vi "MultiPlane.vi"(0 "Digitizer Settings":T5={"Digitizer delay (us) "=0.0, "rf points per line"=2048, "lines per plane"=128, "Samp Rate (Hz)"=100000000.0, "Additional dig delay (us)"=0.0, "Voltage Scale"=0.4, "Pre-Looks"=0, "Offset delay (us)"=0.0, "bits A/D"=8, "Avg Num"=1, "DigTimeOut"=5.0, "Rel Dig Delay"=0.0, "Dig Ch"=0, "LeCroyCluster"={"LeCroy Channels"=[TRUE, FALSE, FALSE, FALSE], "LC read pt offset"=0.0, "Sweep Avg"=FALSE}, "Main Digitizer"=enum."NI Digitizer", "Dig Config"=enum."Single channel", "Digitizer ID Cluster"={"Acqiris/Alazar/SP ID"=[], "NI Instr Handles"=[], "LeCroy VISA"="", "GaGe Handle"={"Handle"=0, "Sample size"=0, "Resolution"=0, "Offset"=0, "Channels"=0, "Boards"=0}, "ATS Ref"="ATS9350", "Acqiris Address"=["PCI::INSTR0"], "ADQRef"=refnum, "adq_cu_ptr"=refnum}, "Trigger Settings"={"Trig Source"=1, "Trig Coupling"=0, "Trig Slope"=0, "Level (mV)"=1500.0}, "Bulk Acq"=FALSE, "Bulk Start Indexes"=[], "Data Ref RF"=refnum, "NI ID/Channel"=[], "Total Dig CH"=5, "Xtra Ann Trig delay (us)"=10.0, "Fix Z Delay?"=FALSE, "One Way Transmission?"=FALSE, "Data Ref Log"=refnum} {"Trigger Settings"."Trig Slope" items=["Positive", "Negative"]; "Trigger Settings"."Level (mV)" format="%.2f"; "Trigger Settings"."Trig Coupling" items=["DC 1 MOhm", "AC 1 MOhm", "DC 50 Ohm", "AC 50 Ohm"]; "Trigger Settings"."Trig Source" items=["Chan 1", "External"]; "Rel Dig Delay" format="%.2f"; "DigTimeOut" format="%.2f"; "Avg Num" min=1; "Offset delay (us)" format="%.2f"; "Additional dig delay (us)" format="%.2f"; "Digitizer delay (us)" format="%.2f"}, 1 "Scan data":T9 {"axis 2 ticks" format="%.2f"; "axis 1 ticks" format="%.2f"; "step size" format="%.2f"; "axis2o" format="%.2f"; "axis1o" format="%.2f"; "Pulse Parameters"."pos peak pressure (MPa)" format="%.2f"; "Pulse Parameters"."focal length (cm)" format="%.2f"; "Pulse Parameters"."MI" format="%.2f"; "Pulse Parameters"."Ita.3" format="%.2f"; "Pulse Parameters"."Temporal Av Intensity \n(Ita mW/cm^2)" format="%.2f"; "Pulse Parameters"."Ipa.3" format="%.2f"; "Pulse Parameters"."Pulse Av Intensity\n (Ipa W/cm^2)" format="%.2f"; "Pulse Parameters"."Pulse Int \nIntegral (PII J/cm^2)" format="%.2f"; "Pulse Parameters"."pulse dur (Pd s)" format="%.2f"; "Pulse Parameters"."p.3" format="%.2f"; "Pulse Parameters"."neg peak pressure (MPa)" format="%.2f"; "Pulse Parameters"."derating (.3) factor" format="%.2f"; "Pulse Parameters"."prf" format="%.2f"; "Pulse Parameters"."Frequency (MHz)" format="%.2f"; "scan data" format="%.2f"}, 3 "Number of z planes":i32=1, 5 "Parameter Selection":u16, 6 "Dig delay":dbl, 7 "Motion Settings":T1={"No Motion?"=FALSE, "Motion System"=enum."No Motion Card", "Motion Bd ID"=1, "Motion Profile"="SMAC1", "# Axis"=1, "Reverse Z axis?"=TRUE, "SMAC Axis"=0, "scan pair"=enum."y-(x) scan", "RT fps"=6.0, "Steps per mm"=[1000, 1000, 1000, 1000], "Motor Parameters"={"velocity ct/s"=[10000.0, 10000.0, 10000.0, 50000.0], "accel ct/s^2"=[50000.0, 50000.0, 50000.0, 200000.0]}, "One Way Scan"=FALSE, "Reverse One Way Scan"=FALSE, "Global Position (mm)"=[], "Plane"=0, "Distance between\nscan lines (um)"=0.0, "Distance between\nscan planes (um)"=0.0, "number of scan planes"=1, "Total steps in line"=0, "Xtra plane\ndistance  (um)"=100, "Xtra planes "=1, "Add Axis"=FALSE, "overshoot cts"=200, "BKPT Shift"=0, "Scan Start Time (ms)"=0, "ESP VISA"="GPIB::1::INSTR", "3rd Axis"=1, "GL Ref Out"=refnum, "Galil Address"=""} {"3rd Axis" items=["x", "y", "z", "w"]; "Xtra planes" min=1; "Xtra plane\ndistance  (um)" min=0; "Distance between\nscan planes (um)" format="%.2f"; "Distance between\nscan lines (um)" format="%.2f"; "SMAC Axis" items=["None"=0, "Axis 1"=1, "Axis 2"=2, "Axis 3"=3, "Axis 4"=4, "Axis 5"=5, "Axis 6"=6, "Axis 7"=7, "Axis 8"=8, "Vector Space 1"=17, "Vector Space 2"=18, "Vector Space 3"=19, "Vector Space 4"=20]; "Motion Bd ID" min=1 max=32 step=1}, 9 "Current plane":i32, 11 "z plane spacing":i32, 12 "file name":string) -> (4 "Digitizer Settings Out":T5={"Digitizer delay (us) "=0.0, "rf points per line"=2048, "lines per plane"=128, "Samp Rate (Hz)"=100000000.0, "Additional dig delay (us)"=0.0, "Voltage Scale"=0.4, "Pre-Looks"=0, "Offset delay (us)"=0.0, "bits A/D"=8, "Avg Num"=1, "DigTimeOut"=5.0, "Rel Dig Delay"=0.0, "Dig Ch"=0, "LeCroyCluster"={"LeCroy Channels"=[TRUE, FALSE, FALSE, FALSE], "LC read pt offset"=0.0, "Sweep Avg"=FALSE}, "Main Digitizer"=enum."NI Digitizer", "Dig Config"=enum."Single channel", "Digitizer ID Cluster"={"Acqiris/Alazar/SP ID"=[], "NI Instr Handles"=[], "LeCroy VISA"="", "GaGe Handle"={"Handle"=0, "Sample size"=0, "Resolution"=0, "Offset"=0, "Channels"=0, "Boards"=0}, "ATS Ref"="ATS9350", "Acqiris Address"=["PCI::INSTR0"], "ADQRef"=refnum, "adq_cu_ptr"=refnum}, "Trigger Settings"={"Trig Source"=1, "Trig Coupling"=0, "Trig Slope"=0, "Level (mV)"=1500.0}, "Bulk Acq"=FALSE, "Bulk Start Indexes"=[], "Data Ref RF"=refnum, "NI ID/Channel"=[], "Total Dig CH"=5, "Xtra Ann Trig delay (us)"=10.0, "Fix Z Delay?"=FALSE, "One Way Transmission?"=FALSE, "Data Ref Log"=refnum} {"Trigger Settings"."Trig Slope" items=["Positive", "Negative"]; "Trigger Settings"."Level (mV)" format="%.2f"; "Trigger Settings"."Trig Coupling" items=["DC 1 MOhm", "AC 1 MOhm", "DC 50 Ohm", "AC 50 Ohm"]; "Trigger Settings"."Trig Source" items=["Chan 1", "External"]; "Rel Dig Delay" format="%.2f"; "DigTimeOut" format="%.2f"; "Avg Num" min=1; "Offset delay (us)" format="%.2f"; "Additional dig delay (us)" format="%.2f"; "Digitizer delay (us)" format="%.2f"}, 15 "Motion Settings Out":T1={"No Motion?"=FALSE, "Motion System"=enum."No Motion Card", "Motion Bd ID"=1, "Motion Profile"="SMAC1", "# Axis"=1, "Reverse Z axis?"=TRUE, "SMAC Axis"=0, "scan pair"=enum."y-(x) scan", "RT fps"=6.0, "Steps per mm"=[1000, 1000, 1000, 1000], "Motor Parameters"={"velocity ct/s"=[10000.0, 10000.0, 10000.0, 50000.0], "accel ct/s^2"=[50000.0, 50000.0, 50000.0, 200000.0]}, "One Way Scan"=FALSE, "Reverse One Way Scan"=FALSE, "Global Position (mm)"=[], "Plane"=0, "Distance between\nscan lines (um)"=0.0, "Distance between\nscan planes (um)"=0.0, "number of scan planes"=1, "Total steps in line"=0, "Xtra plane\ndistance  (um)"=100, "Xtra planes "=1, "Add Axis"=FALSE, "overshoot cts"=200, "BKPT Shift"=0, "Scan Start Time (ms)"=0, "ESP VISA"="GPIB::1::INSTR", "3rd Axis"=1, "GL Ref Out"=refnum, "Galil Address"=""} {"3rd Axis" items=["x", "y", "z", "w"]; "Xtra planes" min=1; "Xtra plane\ndistance  (um)" min=0; "Distance between\nscan planes (um)" format="%.2f"; "Distance between\nscan lines (um)" format="%.2f"; "SMAC Axis" items=["None"=0, "Axis 1"=1, "Axis 2"=2, "Axis 3"=3, "Axis 4"=4, "Axis 5"=5, "Axis 6"=6, "Axis 7"=7, "Axis 8"=8, "Vector Space 1"=17, "Vector Space 2"=18, "Vector Space 3"=19, "Vector Space 4"=20]; "Motion Bd ID" min=1 max=32 step=1})   [LabVIEW 2022 SP3]
uses:
  ScanningControl/Digitizers/-DigitizerRoutines/DigitizerSettings.ctl
  ScanningControl/Digitizers/-DigitizerRoutines/Digitizer.ctl
  ScanningControl/Digitizers/-DigitizerRoutines/DigConfig.ctl
  ScanningControl/Digitizers/-DigitizerRoutines/DigitizerID.ctl
  C:/Windows/System32/ADQAPI_dotNet_helper.dll
  ScanningControl/Motion Controllers/NI_controller/-NI_MotionRoutines/MotionParameters.ctl
  ScanningControl/Motion Controllers/NI_controller/-NI_MotionRoutines/MotionSys.ctl
  ScanningControl/Motion Controllers/-MotionRoutines/ScanAxis.ctl
  ScanningControl/Motion Controllers/-MotionRoutines/3rdAxis.ctl
  ScanningControl/Motion Controllers/-MotionRoutines/MotionGlobals.vi
  <vilib>/Utility/file.llb/Write Delimited Spreadsheet (DBL).vi
panel:
  # "1-D and 2-D B scan settings"
  # "1-D and 2-D B scan settings"
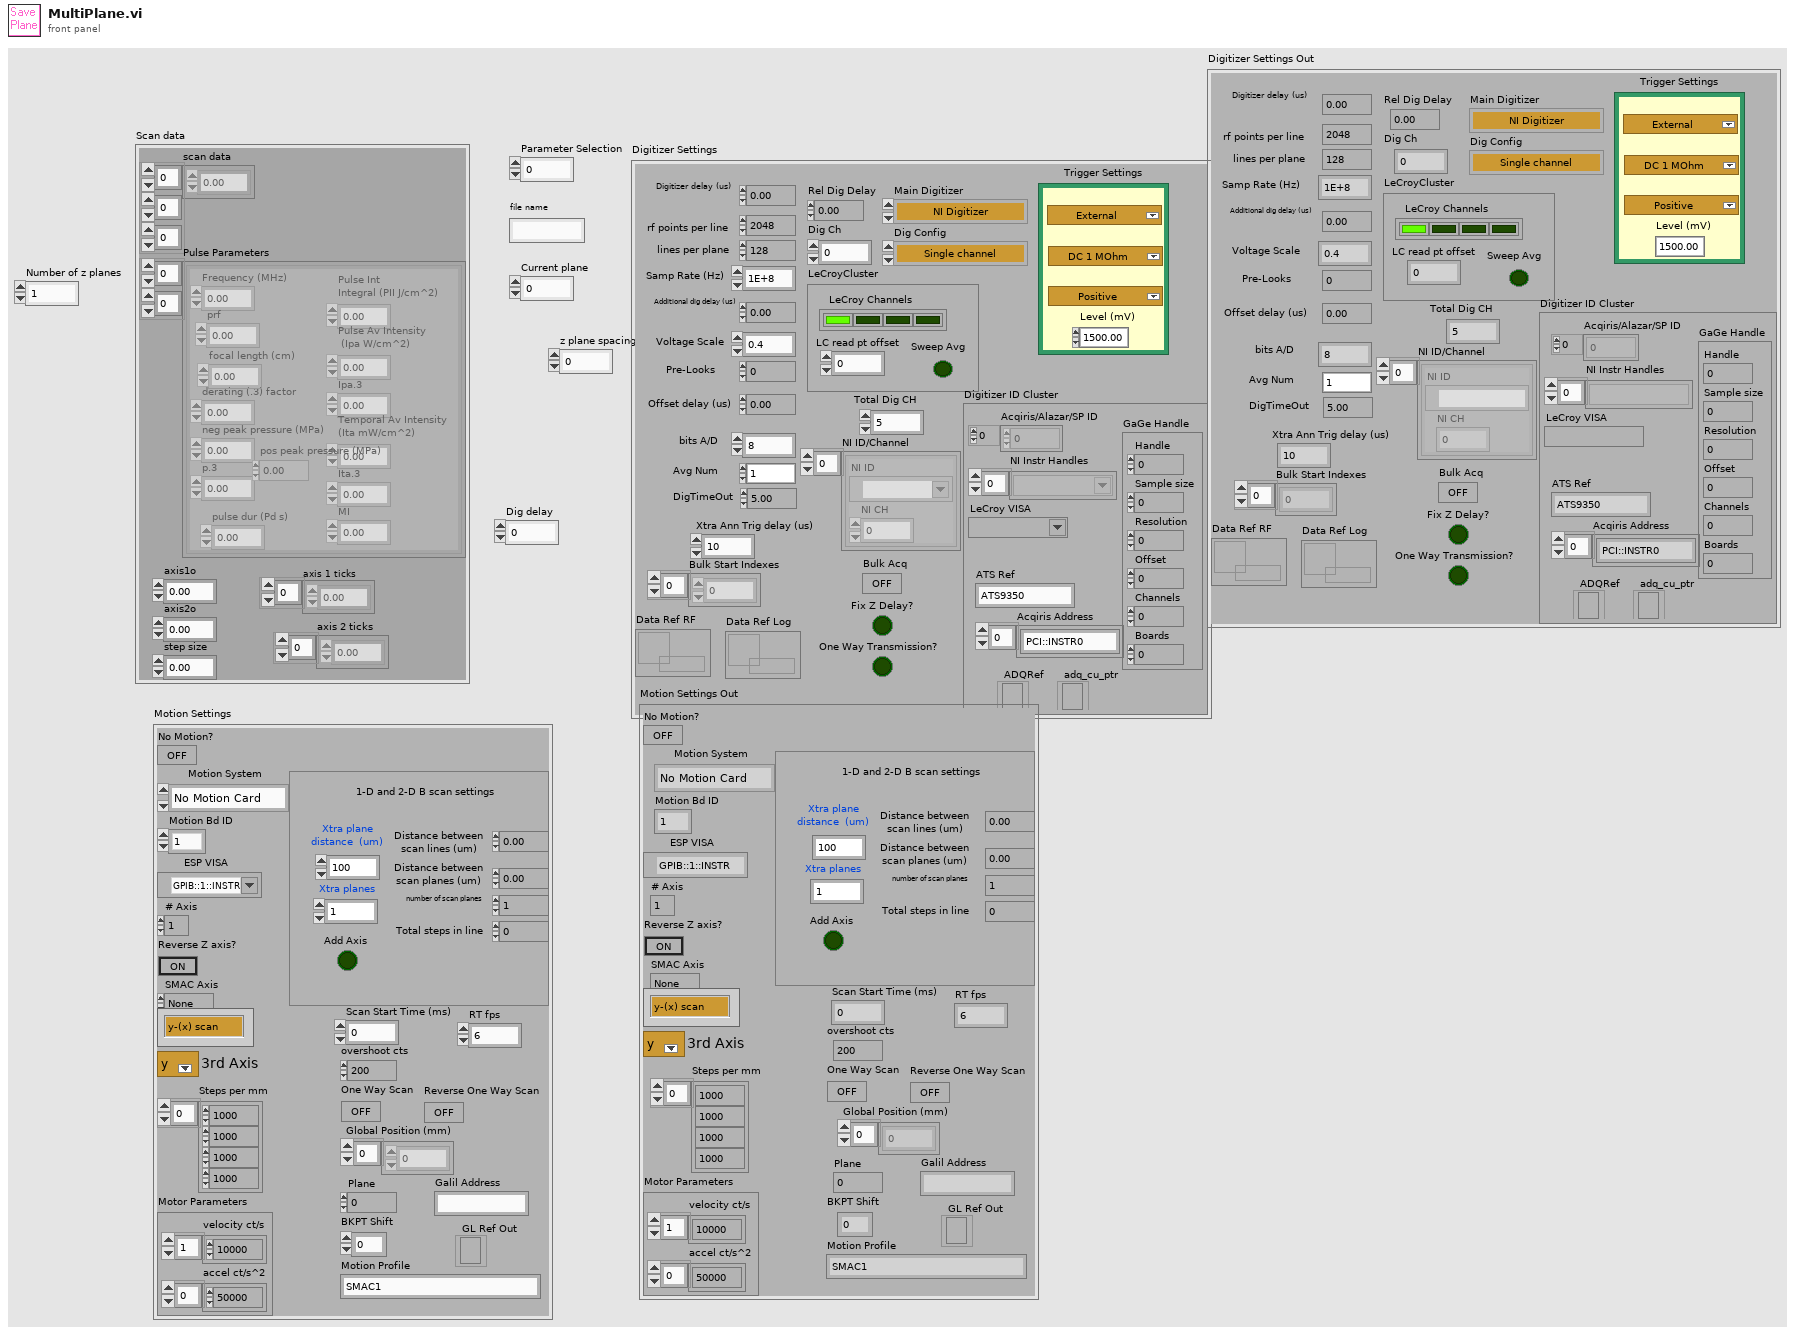
[diagram p1: front panel]
types:
  T1 = typedef "MotionParameters.ctl" = cluster{"No Motion?":bool, "Motion System":T2, "Motion Bd ID":u8, "Motion Profile":string, "# Axis":i8, "Reverse Z axis?":bool, "SMAC Axis":u16, "scan pair":T3, "RT fps":sgl, "Steps per mm":i32[], "Motor Parameters":cluster{"velocity ct/s":dbl[], "accel ct/s^2":dbl[]}, "One Way Scan":bool, "Reverse One Way Scan":bool, "Global Position (mm)":dbl[], "Plane":i32, "Distance between\nscan lines (um)":sgl, "Distance between\nscan planes (um)":sgl, "number of scan planes":i32, "Total steps in line":i32, "Xtra plane\ndistance  (um)":i32, "Xtra planes ":i32, "Add Axis":bool, "overshoot cts":i32, "BKPT Shift":i32, "Scan Start Time (ms)":u32, "ESP VISA":refnum<visa-resource-name>, "3rd Axis":T4, "GL Ref Out":refnum<k7>, "Galil Address":string}
  T2 = typedef "MotionSys.ctl" = enum16{"MM3000", "NI 735x", "Newport ESP", "No Motion Card", "Galil"}
  T3 = typedef "ScanAxis.ctl" = enum16{"y-(x) scan", "x-(y) scan", "z-(x) scan", "z-(y) scan", "y-(z) scan", "x-(z) scan", "w-(x) scan", "w-(y) scan", "w-(z) scan", "x-(w) scan", "y-(w) scan", "z-(w) scan"}
  T4 = typedef "3rdAxis.ctl" = u16
  T5 = typedef "DigitizerSettings.ctl" = cluster{"Digitizer delay (us) ":dbl, "rf points per line":i32, "lines per plane":i32, "Samp Rate (Hz)":dbl, "Additional dig delay (us)":dbl, "Voltage Scale":dbl, "Pre-Looks":i32, "Offset delay (us)":dbl, "bits A/D":i8, "Avg Num":i32, "DigTimeOut":sgl, "Rel Dig Delay":sgl, "Dig Ch":i32, "LeCroyCluster":cluster{"LeCroy Channels":bool[], "LC read pt offset":dbl, "Sweep Avg":bool}, "Main Digitizer":T6, "Dig Config":T7, "Digitizer ID Cluster":T8, "Trigger Settings":cluster{"Trig Source":u16, "Trig Coupling":u16, "Trig Slope":u16, "Level (mV)":dbl}, "Bulk Acq":bool, "Bulk Start Indexes":i32[], "Data Ref RF":refnum<data-value>, "NI ID/Channel":cluster{"NI ID":refnum<k15>, "NI CH":i32}[], "Total Dig CH":i32, "Xtra Ann Trig delay (us)":dbl, "Fix Z Delay?":bool, "One Way Transmission?":bool, "Data Ref Log":refnum<data-value>}
  T6 = typedef "Digitizer.ctl" = enum16{"Acqiris Digitizer", "NI Digitizer", "LeCroy", "GaGe", "AlazarTech", "No Digitizer", "Teledyne"}
  T7 = typedef "DigConfig.ctl" = enum16{"Single channel", "2 Chans w/ 2 Acqiris", "2 Chans w/ 1 Acqiris", "5-CH Pulser New", "5-CH pulser w/ ann array", "5-pass style ann array", "Empty"}
  T8 = typedef "DigitizerID.ctl" = cluster{"Acqiris/Alazar/SP ID":u32[], "NI Instr Handles":refnum<k15>[], "LeCroy VISA":refnum<visa-resource-name>, "GaGe Handle":cluster{"Handle":u32, "Sample size":u32, "Resolution":i32, "Offset":i32, "Channels":u32, "Boards":u32}, "ATS Ref":string, "Acqiris Address":string[], "ADQRef":refnum<k24>, "adq_cu_ptr":refnum<k24>}
  T9 = cluster{"scan data":dbl[][][], "Pulse Parameters":cluster{"Frequency (MHz)":dbl, "prf":dbl, "focal length (cm)":dbl, "derating (.3) factor":dbl, "neg peak pressure (MPa)":dbl, "pos peak pressure (MPa)":dbl, "p.3":dbl, "pulse dur (Pd s)":dbl, "Pulse Int \nIntegral (PII J/cm^2)":dbl, "Pulse Av Intensity\n (Ipa W/cm^2)":dbl, "Ipa.3":dbl, "Temporal Av Intensity \n(Ita mW/cm^2)":dbl, "Ita.3":dbl, "MI":dbl}[][], "axis1o":dbl, "axis2o":dbl, "step size":dbl, "axis 1 ticks":dbl[], "axis 2 ticks":dbl[]}
  T10 = enum16{"Absolute Position", "Relative Position", "Velocity", "Relative to Cap Pos", "Modulus Position", "Absolute Contouring", "Relative Contouring"}
  T11 = typedef "GL Axis Control.ctl" = u16
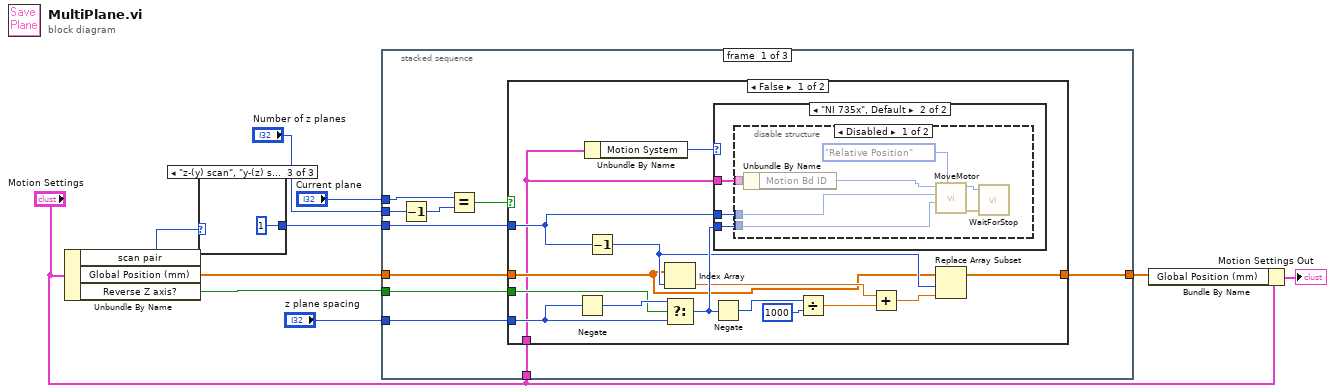
[diagram p0: block diagram]
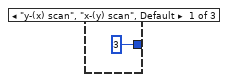
[diagram p2: hidden frame]
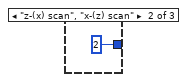
[diagram p3: hidden frame]
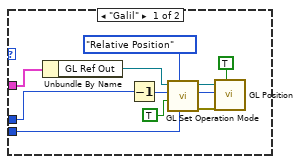
[diagram p4: hidden frame]
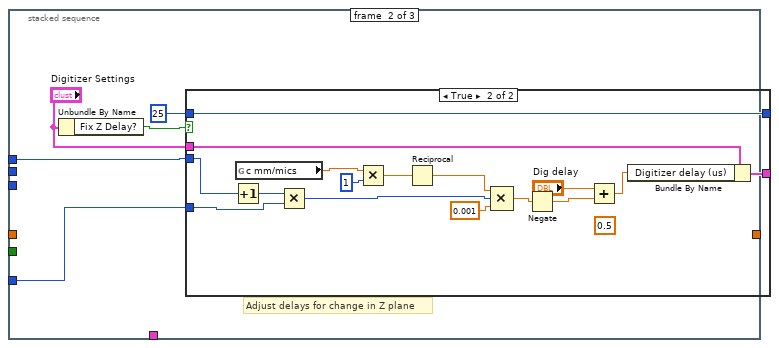
[diagram p7: hidden frame]
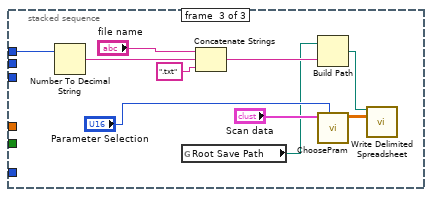
[diagram p9: hidden frame]
diagram:
  n1 = Unbundle By Name("Motion Settings") -> ("scan pair"=w3:T3, "Global Position (mm)"=w7:dbl[], "Reverse Z axis?"=w4:bool)
  n2 = case shown="\"z-(y) scan\", \"y-(z) scan\"" w3 {
    tunnel: [3 2 1] -> w2
    frame "y-(x) scan", "x-(y) scan", Default {
    }
    frame "z-(x) scan", "x-(z) scan" {
    }
    frame "z-(y) scan", "y-(z) scan" {
    }
  }
  n3 = stacked-sequence {
    tunnel: "z plane spacing" -> [w23 w61 _]
    tunnel: "Current plane" -> [w21 w67 w87]
    tunnel: "Number of z planes" -> [w20 _ _]
    tunnel: w7 -> [w18 _ _]
    tunnel: [w17 _ _] -> w5
    tunnel: w4 -> [w16 _ _]
    tunnel: w2 -> [w15 _ _]
    tunnel: "Motion Settings" -> [w14 _ _]
    frame #0 {
      n4 = Decrement(x=w20) -> (x-1=w19:i32)
      n5 = Equal?(x=w21, y=w19) -> (x = y?=w22:bool)
      n6 = case shown="False" w22 {
        tunnel: w23 -> [w33 _]
        tunnel: w18 -> [w29 w60]
        tunnel: [w28 w60] -> w17
        tunnel: w16 -> [w27 _]
        tunnel: w15 -> [w26 _]
        tunnel: w14 -> [w24 _]
        frame False {
          n7 = Negate(x=w33) -> (-x=w38:i32)
          n8 = Unbundle By Name(w24) -> ("Motion System"=w25:T2)
          n9 = Decrement(x=w26) -> (x-1=w32:i32)
          n10 = Index Array(array=w29, index=w32) -> (element=w30:dbl)
          n11 = Select(t=w38, s=w27, f=w33) -> (s? t:f=w35:i32)
          n12 = Negate(x=w35) -> (-x=w34:i32)
          n13 = case shown="\"NI 735x\", Default" w25 {
            tunnel: w26 -> [w42 w52]
            tunnel: w35 -> [w41 w51]
            tunnel: w24 -> [w40 w50]
            frame "Galil" {
              n14 = Unbundle By Name(w40) -> ("GL Ref Out"=w39:refnum<k7>)
              n15 = Decrement(x=w42) -> (x-1=w44:i32)
              n16 = call "GL Set Operation Mode.vi"("position cts (abs/rel)"=w41, "Position Mode (Absolute)"=T10."Relative Position", "Start Now?"=TRUE, "Axis"=w44, "Galil.IGalil"=w39) -> ("error out"=w46:errorcluster, "Axis Out Output"=w45:T11, "Galil Out"=w47:refnum<k7>)  [unwired: 4 in]
              n17 = call "GL Position.vi"("Wait for Motion Complete"=TRUE, "error in (no error)"=w46, "Axis"=w45, "Galil.IGalil"=w47) -> ()  [unwired: 2 in, 4 out]
            }
            frame "NI 735x", Default {
              n18 = disable-structure shown="Disabled" {
                disable-tunnel: w52 -> [w58 _]
                disable-tunnel: w51 -> [w57 _]
                disable-tunnel: w50 -> [w54 _]
                frame Disabled {
                  n19 = Unbundle By Name(w54) -> ("Motion Bd ID"=w53:u8)
                  n20 = call "MoveMotor.vi"("Position Mode (Absolute)"=T10."Relative Position", "Target Position (0)"=w57, "Axis or Vector Space"=w58, "Motion Bd ID"=w53) -> ("error out"=w55:errorcluster, "Bd ID Out"=w56:u8)  [unwired: 1 in, 5 out]
                  n21 = call "WaitForStop.vi"("error in"=w55, "Board ID"=w56) -> ()  [unwired: 4 out]
                }
                frame Enabled {
                }
              }
            }
          }
          n22 = Divide(x=w34, y=1000) -> (x/y=w37:dbl)
          n23 = Add(x=w30, y=w37) -> (x+y=w31:dbl)
          n24 = Replace Array Subset(array=w29, new element=w31, index=w32) -> (w28:dbl[])
        }
        frame True {
        }
      }
    }
    frame #1 {
      # "Adjust delays for change in Z plane"
      n25 = Unbundle By Name("Digitizer Settings") -> ("Fix Z Delay?"=w62:bool)
      n26 = case shown="True" w62 {
        tunnel: w61 -> [_ w79]
        tunnel: w67 -> [_ w78]
        tunnel: [w69 w74] -> w66
        tunnel: 25 -> [w69 w74]
        tunnel: [w68 w73] -> w64
        tunnel: "Digitizer Settings" -> [w68 w72]
        frame False {
        }
        frame True {
          (unwired) 0.5
          n27 = Increment(x=w78) -> (x+1=w77:i32)
          n28 = global read "MotionGlobals.vi" "c mm/mics"() -> (w83:sgl)
          n29 = Multiply(x=w77, y=w79) -> (x*y=w76:i32)
          n30 = Multiply(x=w83, y=1) -> (x*y=w82:sgl)
          n31 = Reciprocal(x=w82) -> (1/x=w84:sgl)
          n32 = Compound Arithmetic op=MULTIPLY(w84, w76, 0.001) -> (w81:dbl)
          n33 = Negate(x=w81) -> (-x=w70:dbl)
          n34 = Add(x="Dig delay", y=w70) -> (x+y=w71:dbl)
          n35 = Bundle By Name(cluster=w72, "Digitizer delay (us)"=w71) -> (w73:T5)
        }
      }
      "Digitizer Settings Out" <- w64
      n36 = Wait (ms)(milliseconds to wait=w66) -> ()  [unwired: 1 out]
    }
    frame #2 {
      n37 = Number To Decimal String(number=w87) -> (decimal integer string=w91:string)  [unwired: 1 out]
      n38 = global read "MotionGlobals.vi" "Root Save Path"() -> (w86:path)
      n39 = Concatenate Strings("file name", w91, ".txt") -> (w94:string)
      n40 = Build Path(base path=w86, name or relative path=w94) -> (appended path=w95:path)
      n41 = call "ChoosePram.vi"("Parameter Selection"="Parameter Selection", "Scan data"="Scan data") -> ("data out"=w90:dbl[][])  [unwired: 2 in, 7 out]
      n42 = call-poly <vilib>:"Write Delimited Spreadsheet.vi"("file path (dialog if empty)"=w95, "2D data"=w90) -> ()  [unwired: 12 in, 2 out]
    }
  }
  n43 = Bundle By Name(cluster="Motion Settings", "Global Position (mm)"=w5) -> (→"Motion Settings Out":T1)
